vi "Construct Terminal Signaling Value Binding.vi"(10 "Ctl Refnum":refnum<vi>) -> (0 "error out":errorcluster, 3 "TerminalSignalingValueBinding":refnum<class "TerminalSignalingValueBinding.lvclass">)   [LabVIEW 2018, in "MVA Framework.lvlib" / "TerminalSignalingValueBinding.lvclass"]
doc: "构建终端信号值绑定"
uses:
  TerminalSignalingValueBinding.lvclass
  <vilib>/Utility/Data Type/NI_Data Type.lvlib
  <vilib>/ErrorRing/Error Ring.xnode
  TerminalPropertyBinding/TerminalPropertyBinding.lvclass
  <vilib>/Utility/error.llb/Error Cluster From Error Code.vi
panel:
  # "Always use TerminalValueBinding unless\nyour code required the signaling effect of\nValue (Signaling) property node write"
  # "除非满足以下条件，否则始终使用TerminalValueBinding\n您的代码需要以下信号效果\n值（信令）属性节点写入"
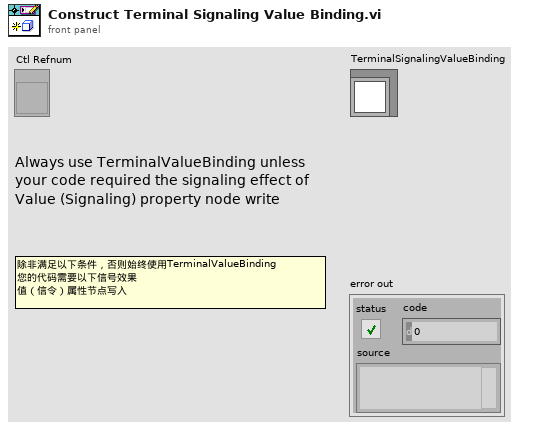
[diagram p1: front panel]
types:
  T1 = typedef "NI_Data Type.lvlib/Data Type.ctl" = enum8{"Invalid Type", "Void", "I8", "I16", "I32", "I64", "U8", "U16", "U32", "U64", "Single Float", "Double Float", "Extended Float", "Single Complex", "Double Complex", "Extended Complex", "Enum U8", "Enum U16", "Enum U32", "Enum U64", "Single Float With Unit", "Double Float With Unit", "Extended Float With Unit", "Single Complex with Unit", "Double Complex with Unit", "Extended Complex with Unit", "Boolean", "String", "Path", "Picture", "Tag", "Array", "Cluster", "Variant", "LV Variant", "Waveform", "Timestamp", "Digital Waveform", "Digital Data", "ExpressData", "Refnum", "External Data", "VI", "Poly VI", "LabVIEW Class Instance", "Fixed Point", "Set Collection", "Map Collection"}
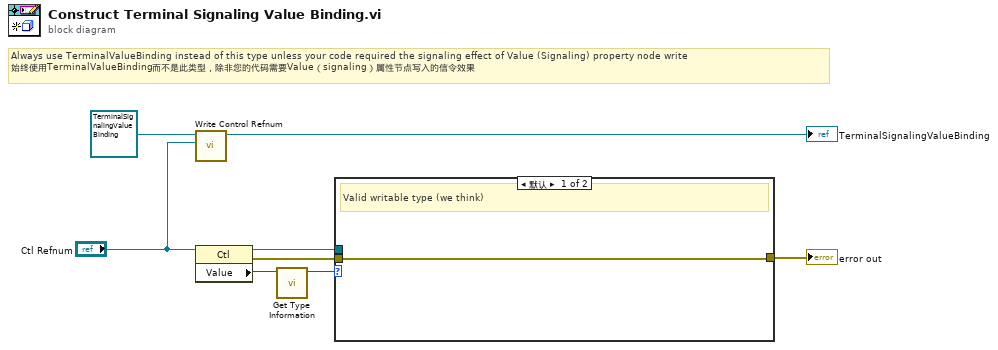
[diagram p0: block diagram]
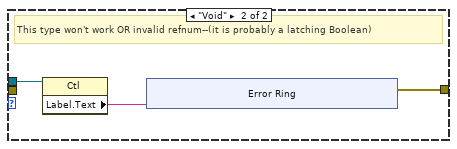
[diagram p2: hidden frame]
diagram:
  # "Always use TerminalValueBinding instead of this type unless your code required the signaling effect of Value (Signaling) property node write\n始终使用TerminalValueBinding而不是此类型，除非您的代码需要Value（signaling）属性节点写入的信令效果"
  n1 = call "Write Control Refnum.vi"("Ctl Refnum"="Ctl Refnum", "TerminalReference in"=refnum<class "TerminalSignalingValueBinding.lvclass"> refnum) -> ("TerminalReferenceBinding Out"=→"TerminalSignalingValueBinding":refnum<class "TerminalSignalingValueBinding.lvclass">)  [unwired: 9 in]
  n2 = property class="Ctl"(reference="Ctl Refnum") -> (reference out=w5:refnum<vi>, error out=w4:errorcluster, "Value"=w8:variant)  [unwired: 1 in]
  n3 = call <vilib>:"Get Type Information.vi"("variant"=w8) -> ("type"=w6:T1)  [unwired: 6 in, 4 out]
  n4 = case shown="默认" w6 {
    tunnel: w5 -> [_ w12]
    tunnel: w4 -> [w9 _]
    tunnel: [w9 w10] -> w3
    frame Default {
      # "Valid writable type (we think)"
    }
    frame "Void" {
      # "This type won't work OR invalid refnum--(it is probably a latching Boolean)"
      n5 = property class="Ctl"(reference=w12) -> ("Label.Text"=w11:string)  [unwired: 1 in, 2 out]
      n6 = xnode "Error Ring"("参数 0"=w11) -> ("错误输出"=w10:errorcluster)
    }
  }
  "error out" <- w3
